vi "transActForceCoorSys.vi"(8 "error in (no error)":errorcluster, 10 "Actuator Force (N)":dbl[](array[numeric]), 11 "SubSysAdap in":refnum<class "SubSysAdap.lvclass">) -> (0 "error out":errorcluster, 2 "Transformed Actuator Force (N)":dbl[](array[numeric]), 3 "SubSysAdap out":refnum<class "SubSysAdap.lvclass">)   [LabVIEW 2016, in "OfcFunc.lvlib" / "SubSysAdap.lvclass"]
doc: "Transform the actuator force between the Zemax coordinate system and the mirror coordinate system."
uses:
  SubSysAdap.lvclass
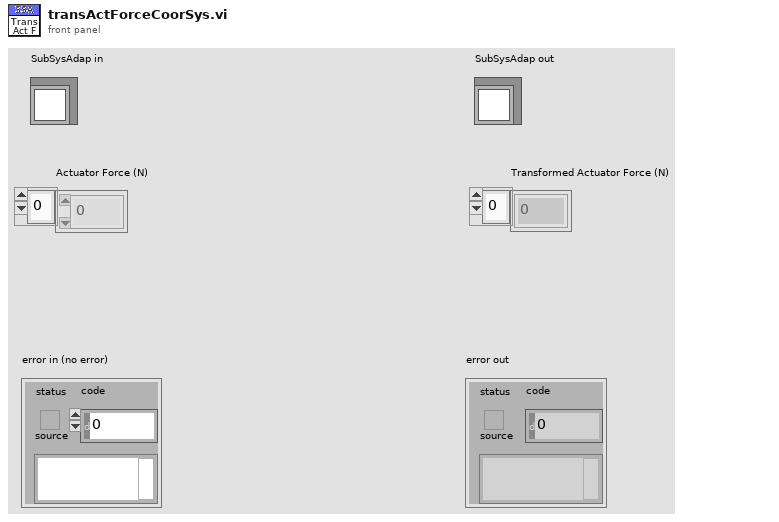
[diagram p1: front panel]
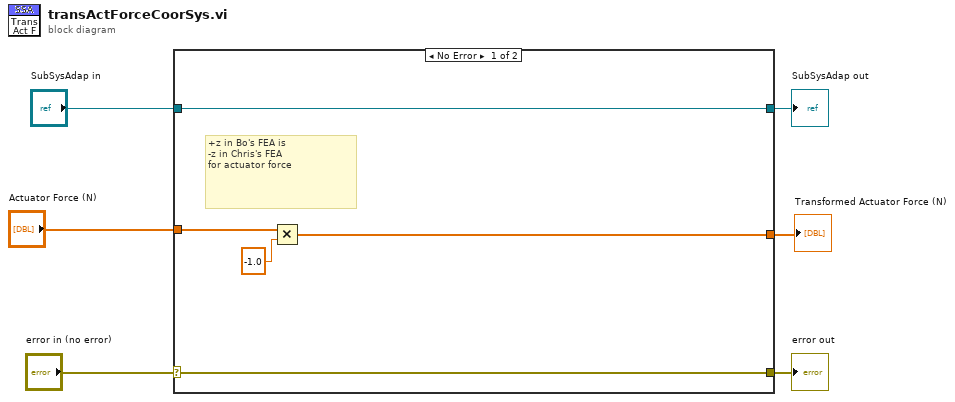
[diagram p0: block diagram]
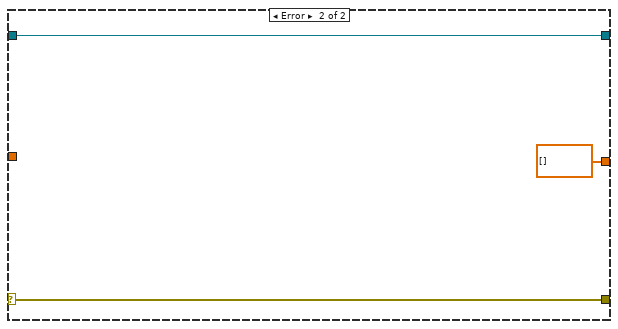
[diagram p2: hidden frame]
diagram:
  n1 = case shown="No Error" "error in (no error)" {
    selector: "error in (no error)" -> [w10 w14]
    tunnel: [w10 w14] -> w5
    tunnel: [w11 w13] -> w3
    tunnel: "SubSysAdap in" -> [w11 w13]
    tunnel: "Actuator Force (N)" -> [w8 _]
    tunnel: [w7 dbl[] []] -> w1
    frame No Error {
      # "+z in Bo's FEA is \n-z in Chris's FEA\nfor actuator force"
      n2 = Multiply(x=w8, y=-1.0 ("Numeric")) -> (x*y=w7:dbl[])
    }
    frame Error {
    }
  }
  "error out" <- w5
  "SubSysAdap out" <- w3
  "Transformed Actuator Force (N)" <- w1
